vi "Update UI per Reference.vi"(8 "error in (no error)":errorcluster, 11 "Analyze Results Beam Deviation in":refnum<class "Analyze Results Beam Deviation.lvclass">) -> (0 "error out":errorcluster, 3 "Analyze Results Beam Deviation out":refnum<class "Analyze Results Beam Deviation.lvclass">)   [LabVIEW 2020, in "Analyze Results Beam Deviation.lvclass"]
uses:
  Analyze Results Beam Deviation.lvclass
  Analyze Results Beam Deviation.lvclass/Analyze Results Beam Deviation.ctl
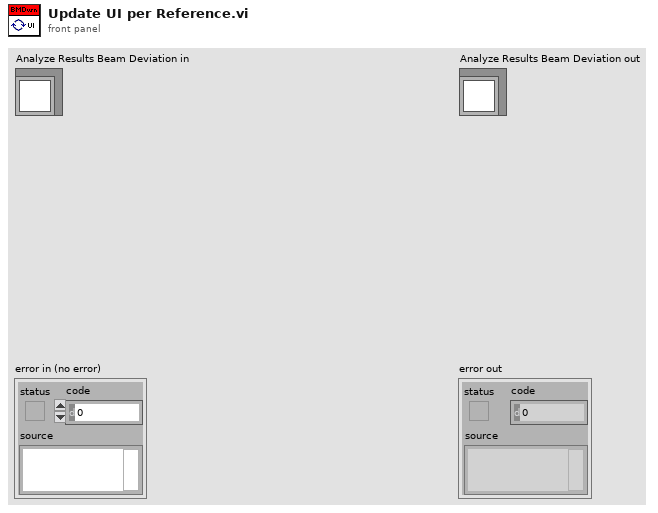
[diagram p1: front panel]
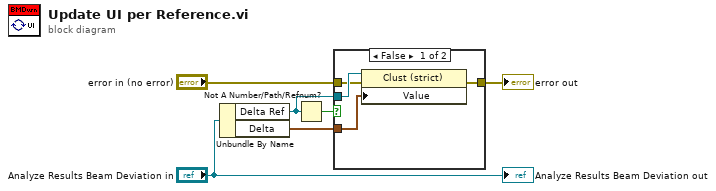
[diagram p0: block diagram]
diagram:
  n1 = Unbundle By Name("Analyze Results Beam Deviation in") -> ("Delta Ref"=w2:refnum<vi>, "Delta"=w6:cluster{"x":sgl, "y":sgl})
  n2 = Not A Number/Path/Refnum?(number/path/refnum=w2) -> (NaN/Path/Refnum?=w1:bool)
  n3 = case shown="False" w1 {
    tunnel: w2 -> [w10 _]
    tunnel: w6 -> [w9 _]
    tunnel: "error in (no error)" -> [w8 w11]
    tunnel: [w7 w11] -> w3
    frame False {
      n4 = property class="Clust (strict)"(reference=w10, error in=w8, "Value"=w9) -> (error out=w7:errorcluster)  [unwired: 1 out]
    }
    frame True {
    }
  }
  "error out" <- w3
  "Analyze Results Beam Deviation out" <- "Analyze Results Beam Deviation in"
